vi "LCOS GUI v3_red.vi"() -> ()   [LabVIEW 2011]
uses:
  Periodic Spot Pattern Parameters.ctl
  LCOS State Machine States.ctl
  LCOS Pattern Display Actions.ctl
  LCOS Parent Action.ctl
  LCOS Images.ctl
  <vilib>/vision/Image Controls.llb/IMAQ Image.ctl
panel:
  in  "Enable Remote Control":bool=TRUE
  in  "Clear Error":bool
  in  "Ignore":bool
  out "Last Error":errorcluster
  in  "Loaded Pattern File:":bool
  out "File Path":path
  out "LCOS Pattern Preview":T1(plugin-control)
  in  "Buttons":T2={"Pattern"=enum."Computed", "Auto-Update LCOS"=TRUE, "Apply Correction"=FALSE, "Update LCOS"=FALSE, "Preview Pattern"=FALSE, "Auto-Preview"=TRUE}
  in  "Pattern Definition":T3={"X pitch"=23.0, "rotation"=0.0, "Center H"=0.0, "Center V"=0.0, "# Spots H"=5, "# Spots V"=13, "Spot size"=23.0, "ref_spot _dark"=FALSE, "Exact Phase Formula"=TRUE, "phase_wrap_pos"=FALSE, "Set Focus (mm)"=32.0, "phase_max"=4.0, "phase_factor"=60, "Steer LW"=1, "Steer vmax"=80, "phase_wrap_neg"=TRUE, "steer_horiz"=FALSE, "steer_pad"=0, "steer_only"=FALSE, "Wavelength"=6.28e-07, "Y pitch"=23.0, "python"=TRUE, "test_pattern"=FALSE, "grid"=TRUE, "dark_all"=FALSE, "Xm_str"="21.72,  44.87,  68.20,  91.45, 114.72, 137.87, 160.97, 184.04", "Ym_str"="21.72,  44.87,  68.20,  91.45, 114.72, 137.87, 160.97, 184.04", "ref_spot"=0, "stretch"=TRUE} {"ref_spot" min=0 max=500 step=1 format="%#.0f"; "Y pitch" min=0.0 max=100.0 format="%.2g"; "Wavelength" min=0.0 max=500.0 format="%^#.3e"; "steer_pad" min=0 max=500 step=1 format="%#.0f"; "Steer LW" max=500; "phase_max" min=0.0 max=500.0 format="%#.3f"; "Set Focus (mm)" min=0.0 max=500.0 format="%#.3g"; "Spot size" min=1.0 format="%.2g"; "# Spots V" min=1 step=1; "# Spots H" min=1 step=1; "Center V" format="%.2f"; "Center H" format="%.2f"; "rotation" min=-90.0 max=90.0 format="%.2g"; "X pitch" min=0.0 max=100.0 format="%.2g"}
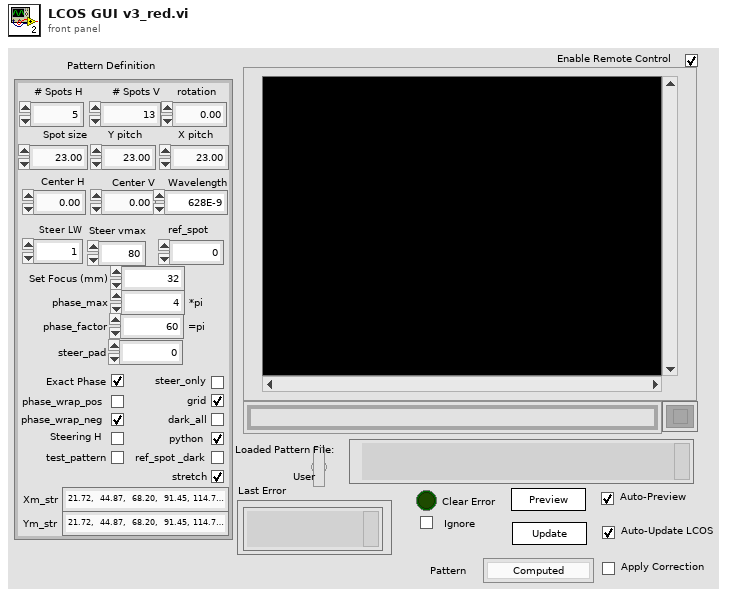
[diagram p1: front panel]
types:
  T1 = typedef "IMAQ Image.ctl" = refnum<image>
  T2 = cluster{"Pattern":enum16{"Computed", "From File", "Correction"}, "Auto-Update LCOS":bool, "Apply Correction":bool, "Update LCOS":bool, "Preview Pattern":bool, "Auto-Preview":bool}
  T3 = typedef "Periodic Spot Pattern Parameters.ctl" = cluster{"X pitch":dbl, "rotation":dbl, "Center H":dbl, "Center V":dbl, "# Spots H":u32, "# Spots V":u32, "Spot size":dbl, "ref_spot _dark":bool, "Exact Phase Formula":bool, "phase_wrap_pos":bool, "Set Focus (mm)":dbl, "phase_max":dbl, "phase_factor":u8, "Steer LW":u32, "Steer vmax":u8, "phase_wrap_neg":bool, "steer_horiz":bool, "steer_pad":i64, "steer_only":bool, "Wavelength":dbl, "Y pitch":dbl, "python":bool, "test_pattern":bool, "grid":bool, "dark_all":bool, "Xm_str":string, "Ym_str":string, "ref_spot":i64, "stretch":bool}
  T4 = typedef "LCOS Pattern Display Actions.ctl" = enum16{"Init", "Idle", "Update", "Exit"}
  T5 = cluster{"LCOS Pattern Display Actions":T4, "Data":variant}
  T6 = typedef "LCOS State Machine States.ctl" = enum16{"Init", "Idle", "Preview Button Pushed", "Update Button Pushed", "Pattern Selection Changed", "Pattern Definition Changed", "Selected File Changed", "Load Correction Pattern", "Load Correction Pattern Step 2", "Load User Pattern", "Load User Pattern Step 2", "Compute Pattern", "Correct Pattern", "Update Preview Display", "Update LCOS Display", "Error", "Clear Error", "Exit"}
  T7 = cluster{"X pitch":dbl, "rotation":dbl, "Center H":dbl, "Center V":dbl, "# Spots H":u32, "# Spots V":u32, "Spot size":dbl, "ref_spot _dark":bool, "Exact Phase Formula":bool, "phase_wrap_pos":bool, "Set Focus (mm)":dbl, "phase_max":dbl, "phase_factor":u8, "Steer LW":u32, "Steer vmax":u8, "phase_wrap_neg":bool, "steer_horiz":bool, "steer_pad":i64, "steer_only":bool, "Wavelength":dbl, "Y pitch":dbl, "python":bool, "test_pattern":bool, "grid":bool, "dark_all":bool, "Xm_str":string, "Ym_str":string, "ref_spot":i64, "stretch":bool}
  T8 = typedef "LCOS Parent Action.ctl" = enum16{"Pattern Definition Changed", "Preview Button Pushed", "Update Button Pushed", "Pattern Selection Changed", "Correction Pattern Changed", "User Pattern (from File) Changed"}
  T9 = typedef "LCOS Images.ctl" = cluster{"Computed Pattern Image":T1, "User Pattern (from File) Image":T1, "Correction Pattern Image":T1, "Corrected Pattern Image":T1, "Preview Image":T1, "LCOS Displayed Image":T1}
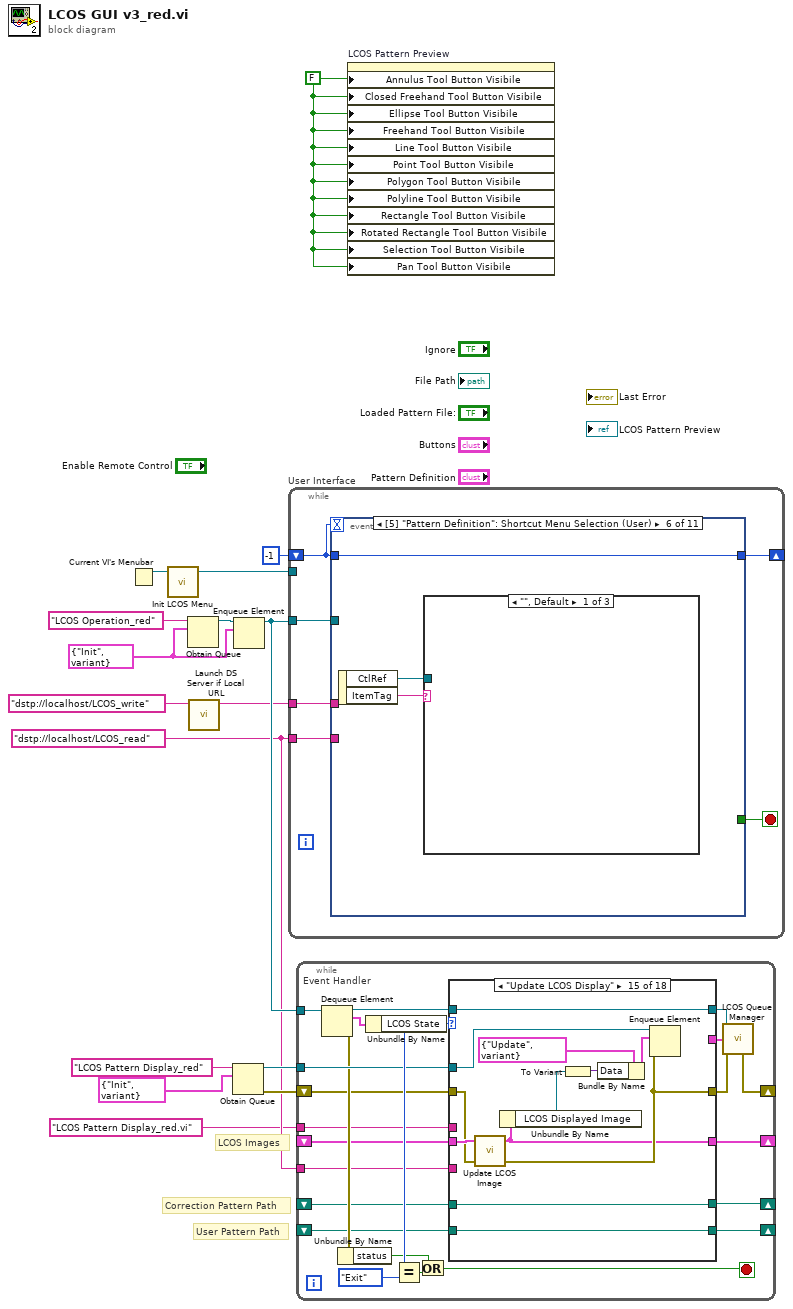
[diagram p0: block diagram]
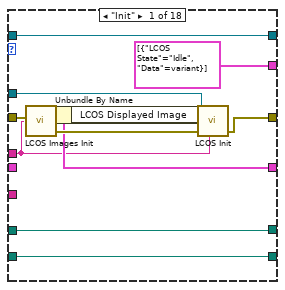
[diagram p2: hidden frame]
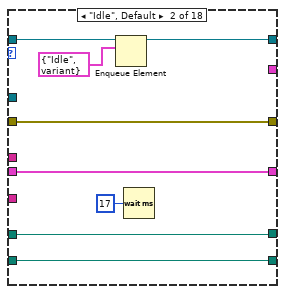
[diagram p3: hidden frame]
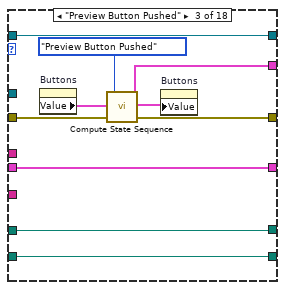
[diagram p4: hidden frame]
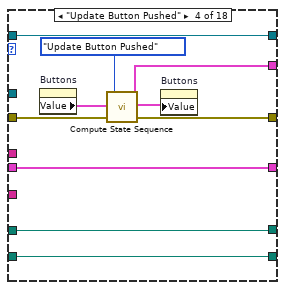
[diagram p5: hidden frame]
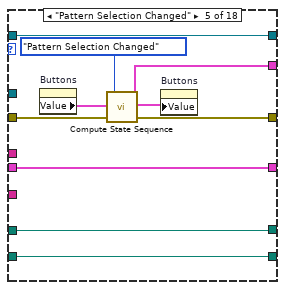
[diagram p6: hidden frame]
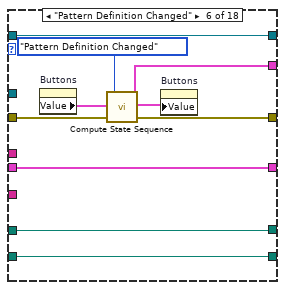
[diagram p7: hidden frame]
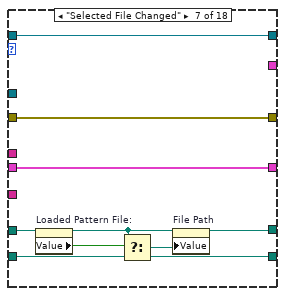
[diagram p8: hidden frame]
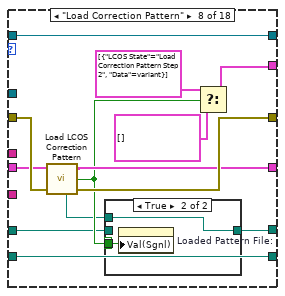
[diagram p9: hidden frame]
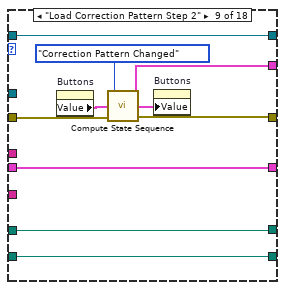
[diagram p11: hidden frame]
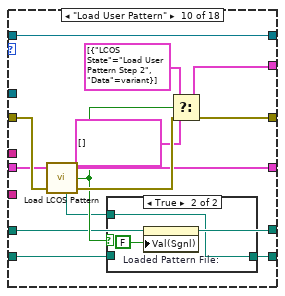
[diagram p12: hidden frame]
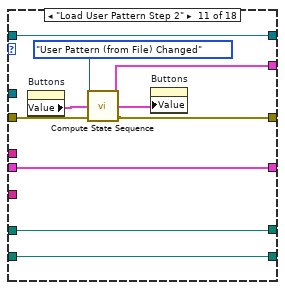
[diagram p14: hidden frame]
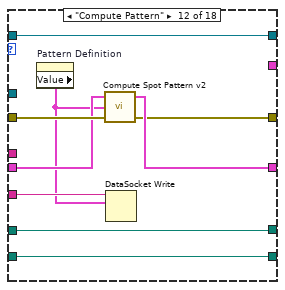
[diagram p15: hidden frame]
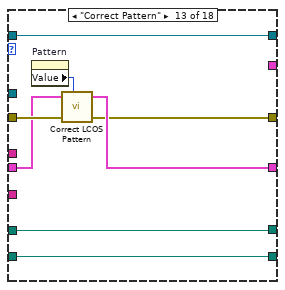
[diagram p16: hidden frame]
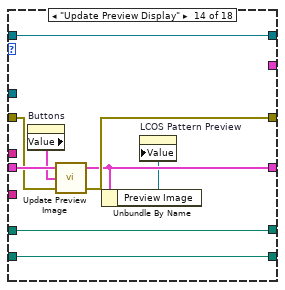
[diagram p17: hidden frame]
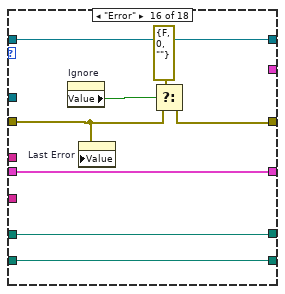
[diagram p18: hidden frame]
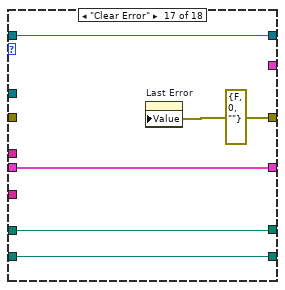
[diagram p19: hidden frame]
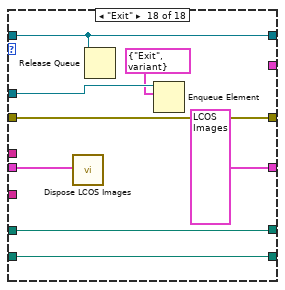
[diagram p20: hidden frame]
diagram:
  w2 = "dstp://localhost/LCOS_read" ("URL")
  w6 = FALSE ("ROI Tool Buttons Visibile:Annulus Tool Button Visibile")
  w7 = cluster{"LCOS State":T6, "Data":variant} {"LCOS State"=enum."Init", "Data"=variant}
  # "User Pattern Path"
  # "Correction Pattern Path"
  # "LCOS Images"
  n1 = Current VI's Menubar() -> (w16:refnum<k9>)
  n2 = call "Init LCOS Menu.vi"("Menu Refnum (in)"=w16) -> ("Menu Refnum (out)"=w15:refnum<k9>)  [unwired: 7 in, 1 out]
  n3 = Obtain Queue(name (unnamed)="LCOS Operation_red", element data type=w7) -> (queue out=w9:refnum<queue>)  [unwired: 3 in, 2 out]
  n4 = call "Launch DS Server if Local URL.vi"("URL"="dstp://localhost/LCOS_write") -> ("Duplicate URL"=w3:string)  [unwired: 5 in, 1 out]
  n5 = Obtain Queue(name (unnamed)="LCOS Pattern Display_red", element data type=T5 {"LCOS Pattern Display Actions"=enum."Init", "Data"=variant}) -> (queue out=w11:refnum<queue>, error out=w10:errorcluster)  [unwired: 3 in, 1 out]
  n6 = Enqueue Element(queue=w9, element=w7) -> (queue out=w8:refnum<queue>)  [unwired: 2 in, 2 out]
  n7 = while "User Interface" {
    tunnel: w15 -> [_]
    tunnel: w8 -> [w21]
    shift-right: [w20] -> _
    shift-left: -1 -> [w19]
    tunnel: w3 -> [w18]
    tunnel: w2 -> [w17]
    stop <- w22 stop-if-true
    n8 = event shown="[5] \"Pattern Definition\": Shortcut Menu Selection (User)" {
      selector: _ -> [_ _ _ _ _ _ _ _ _ _ _]
      dyn-events: _ -> [_ _ _ _ _ _ _ _ _ _ _]
      timeout: w19 -> [_ _ _ _ _ _ _ _ _ _ _]
      tunnel: [_ _ _ _ _ _ _ _ _ w63 w81] -> w22
      tunnel: w21 -> [_ _ w41 w44 w47 _ w55 w58 w61 w64 w80]
      tunnel: [w23 w35 w39 w42 w45 w50 w53 w56 w59 w62 w78] -> w20
      tunnel: w19 -> [w23 _ w39 w42 w45 w50 w53 w56 w59 w62 w78]
      tunnel: w18 -> [w28 _ _ _ _ _ _ _ _ _ _]
      tunnel: w17 -> [w24 w32 _ _ _ _ _ _ _ _ _]
      event Timeout {
        n9 = event-data() -> ()  [unwired: 1 in, 1 out]
        n10 = DataSocket Read(9:w23, 10:T3 {"X pitch"=0.0, "rotation"=0.0, "Center H"=0.0, "Center V"=0.0, "# Spots H"=0, "# Spots V"=0, "Spot size"=0.0, "ref_spot _dark"=FALSE, "Exact Phase Formula"=FALSE, "phase_wrap_pos"=FALSE, "Set Focus (mm)"=0.0, "phase_max"=0.0, "phase_factor"=0, "Steer LW"=0, "Steer vmax"=0, "phase_wrap_neg"=FALSE, "steer_horiz"=FALSE, "steer_pad"=0, "steer_only"=FALSE, "Wavelength"=0.0, "Y pitch"=0.0, "python"=FALSE, "test_pattern"=FALSE, "grid"=FALSE, "dark_all"=FALSE, "Xm_str"="", "Ym_str"="", "ref_spot"=0, "stretch"=FALSE} ("Pattern Definition"), 11:w28) -> (1:w26:bool, 2:w25:T3)  [unwired: 2 in, 5 out]
        n11 = case shown="False" w26 {
          tunnel: w25 -> [w30 _]
          tunnel: w24 -> [w31 _]
          tunnel: w23 -> [w29 _]
          frame False {
            n12 = property on="Pattern Definition" class="Clust (strict)"("Val(Sgnl)"=w30) -> ()  [unwired: 2 in, 2 out]
            n13 = DataSocket Write(9:w29, 10:w30, 11:w31) -> ()  [unwired: 1 in, 3 out]
          }
          frame True {
          }
        }
      }
      event "Enable Remote Control": Value Change {
        n14 = event-data() -> ("NewVal"=w33:bool)  [unwired: 1 in]
        n15 = case shown="False" w33 {
          tunnel: w32 -> [_ w38]
          frame False {
          }
          frame True {
            n16 = property on="Pattern Definition" class="Clust (strict)"() -> ("Value"=w37:T7)  [unwired: 2 in, 2 out]
            n17 = DataSocket Write(10:w37, 11:w38) -> ()  [unwired: 2 in, 3 out]
          }
        }
        n18 = Select(t=1, s=w33, f=-1) -> (s? t:f=w35:i32)
      }
      event Value Change {
        n19 = event-data() -> ()  [unwired: 1 in, 1 out]
        n20 = Enqueue Element(queue=w41, element=cluster{"LCOS State":T6, "Data":variant} {"LCOS State"=enum."Pattern Definition Changed", "Data"=variant}) -> ()  [unwired: 2 in, 3 out]
      }
      event "Buttons.Preview Pattern": Value Change {
        n21 = event-data() -> ()  [unwired: 1 in, 1 out]
        n22 = Enqueue Element(queue=w44, element=cluster{"LCOS State":T6, "Data":variant} {"LCOS State"=enum."Preview Button Pushed", "Data"=variant}) -> ()  [unwired: 2 in, 3 out]
      }
      event "Buttons.Update LCOS": Value Change {
        n23 = event-data() -> ()  [unwired: 1 in, 1 out]
        n24 = Enqueue Element(queue=w47, element=cluster{"LCOS State":T6, "Data":variant} {"LCOS State"=enum."Update Button Pushed", "Data"=variant}) -> ()  [unwired: 2 in, 3 out]
      }
      event Shortcut Menu Selection (User) {
        n25 = event-data() -> ("CtlRef"=w48:refnum<vi>, "ItemTag"=w49:string)  [unwired: 1 in]
        n26 = case shown="\"\", Default" w49 {
          tunnel: w48 -> [_ w51 w52]
          frame "", Default {
          }
          frame "Save Configuration" {
            n27 = call "Save LCOS Configuration.vi"("LCOS Configuration Ref"=w51) -> ()  [unwired: 11 in]
          }
          frame "Load Configuration" {
            n28 = call "Load LCOS Configuration.vi"("LCOS Configuration Ref"=w52) -> ()  [unwired: 11 in]
          }
        }
      }
      event "Buttons.Pattern": Value Change {
        n29 = event-data() -> ()  [unwired: 1 in, 4 out]
        n30 = Enqueue Element(queue=w55, element=cluster{"LCOS State":T6, "Data":variant} {"LCOS State"=enum."Pattern Selection Changed", "Data"=variant}) -> ()  [unwired: 2 in, 3 out]
      }
      event "Clear Error": Value Change {
        n31 = event-data() -> ()  [unwired: 1 in, 1 out]
        n32 = Enqueue Element(queue=w58, element=cluster{"LCOS State":T6, "Data":variant} {"LCOS State"=enum."Clear Error", "Data"=variant}) -> ()  [unwired: 2 in, 3 out]
      }
      event "Loaded Pattern File:": Value Change {
        n33 = event-data() -> ()  [unwired: 1 in, 1 out]
        n34 = Enqueue Element(queue=w61, element=cluster{"LCOS State":T6, "Data":variant} {"LCOS State"=enum."Selected File Changed", "Data"=variant}) -> ()  [unwired: 2 in, 3 out]
      }
      event Menu Selection (User) {
        n35 = event-data() -> ("ItemTag"=w65:string)  [unwired: 1 in]
        n36 = case shown="\"Load Correction Pattern\"" w65 {
          tunnel: w64 -> [_ w67 w69 w73]
          tunnel: [_ _ _ w70] -> w63
          frame "-", Default {
          }
          frame "Load Correction Pattern" {
            n37 = Enqueue Element(queue=w67, element=cluster{"LCOS State":T6, "Data":variant} {"LCOS State"=enum."Load Correction Pattern", "Data"=variant}) -> ()  [unwired: 2 in, 3 out]
          }
          frame "Load User Pattern" {
            n38 = Enqueue Element(queue=w69, element=cluster{"LCOS State":T6, "Data":variant} {"LCOS State"=enum."Load User Pattern", "Data"=variant}) -> ()  [unwired: 2 in, 3 out]
          }
          frame "Quit" {
            n39 = Two Button Dialog(message="Do you want to quit?") -> (T button?=w70:bool)  [unwired: 2 in]
            n40 = case shown="True" w70 {
              tunnel: w73 -> [w74 w77]
              tunnel: [w74 w76] -> _
              tunnel: cluster{"LCOS State":T6, "Data":variant} {"LCOS State"=enum."Exit", "Data"=variant} ("element") -> [_ w75]
              frame False {
              }
              frame True {
                n41 = Enqueue Element(queue=w77, element=w75) -> (queue out=w76:refnum<queue>)  [unwired: 2 in, 2 out]
              }
            }
          }
        }
      }
      event Panel Close? {
        w81 = TRUE ("Discard?")
        n42 = event-data() -> ()  [unwired: 1 in, 1 out]
        n43 = Enqueue Element(queue=w80, element=cluster{"LCOS State":T6, "Data":variant} {"LCOS State"=enum."Exit", "Data"=variant}) -> ()  [unwired: 2 in, 3 out]
        n44 = event-data("Discard?"=w81) -> ()  [unwired: 1 in, 1 out]
      }
    }
  }
  n45 = while "Event Handler" {
    tunnel: w11 -> [w99]
    shift-right: [w93] -> _
    shift-left: w10 -> [w91]
    tunnel: w8 -> [w104]
    shift-right: [w89] -> _
    shift-left: _ -> [w90]
    shift-right: [w87] -> _
    shift-left: _ -> [w86]
    shift-right: [w85] -> _
    shift-left: _ -> [w84]
    tunnel: w2 -> [w83]
    tunnel: "LCOS Pattern Display_red.vi" ("name (unnamed)") -> [w82]
    stop <- w96 stop-if-true
    n46 = Dequeue Element(queue=w104) -> (queue out=w100:refnum<queue>, element=w98:cluster{"LCOS State":T6, "Data":variant}, error out=w97:errorcluster)  [unwired: 2 in, 1 out]
    n47 = Unbundle By Name(w97) -> ("status"=w95:bool)
    n48 = Unbundle By Name(w98) -> ("LCOS State"=w103:T6)
    n49 = Equal?(x=w103, y=LCOS_State_Machine_States."Exit") -> (x = y?=w101:bool)
    n50 = Or(x=w95, y=w101) -> (x .or. y?=w96:bool)
    n51 = case shown="\"Update LCOS Display\"" w103 {
      tunnel: w100 -> [w108 w123 w130 w140 w150 w160 w170 w178 w194 w204 w220 w227 w234 w248 w256 w263 w271 w276]
      tunnel: w99 -> [w115 _ _ _ _ _ _ _ _ _ _ _ _ _ w260 _ _ w280]
      tunnel: [cluster{"LCOS State":T6, "Data":variant}[] [{"LCOS State"=enum."Idle", "Data"=variant}] ("Action Sequence") _ w127 w137 w147 w157 _ w181 w191 w206 w217 _ _ _ _ _ _ _] -> w94
      tunnel: [w114 w121 w128 w138 w148 w158 w169 w182 w192 w208 w218 w228 w235 w244 w253 w266 w273 w281] -> w92
      tunnel: w91 -> [w113 w121 w129 w139 w149 w159 w169 w183 w193 w209 w219 w231 w238 w245 w254 w264 _ w281]
      tunnel: w90 -> [_ w119 w132 w142 w152 w162 w168 w177 w189 w203 w215 w230 w237 w247 w255 w268 w272 w278]
      tunnel: [w110 w119 w132 w142 w152 w162 w168 w176 w189 w202 w215 w229 w236 w243 w252 w268 w272 T9 {"Computed Pattern Image"=refnum, "User Pattern (from File) Image"=refnum, "Correction Pattern Image"=refnum, "Corrected Pattern Image"=refnum, "Preview Image"=refnum, "LCOS Displayed Image"=refnum} ("Images")] -> w89
      tunnel: [w108 w118 w130 w140 w150 w160 w170 w178 w194 w204 w220 w227 w234 w248 w256 w263 w271 w276] -> w88
      tunnel: [w107 w117 w125 w135 w145 w155 w165 w173 w188 w197 w214 w226 w233 w241 w250 w262 w270 w275] -> w87
      tunnel: w86 -> [w107 w117 w125 w135 w145 w155 w165 w174 w188 w197 w214 w226 w233 w241 w250 w262 w270 w275]
      tunnel: [w106 w116 w124 w134 w144 w154 w166 w171 w187 w199 w213 w225 w232 w240 w249 w261 w269 w274] -> w85
      tunnel: w84 -> [w106 w116 w124 w134 w144 w154 w166 w171 w187 w198 w213 w225 w232 w240 w249 w261 w269 w274]
      tunnel: w83 -> [_ _ _ _ _ _ _ _ _ _ _ w224 _ _ _ _ _ _]
      tunnel: w82 -> [w105 _ _ _ _ _ _ _ _ _ _ _ _ _ _ _ _ _]
      frame "Init" {
        n52 = call "LCOS Images Init.vi"("LCOS Pattern Display.vi Name"=w105, "error in (no error)"=w113) -> ("Images"=w110:T9, "error out"=w112:errorcluster)  [unwired: 6 in]
        n53 = Unbundle By Name(w110) -> ("LCOS Displayed Image"=w111:T1)
        n54 = call "LCOS Init.vi"("LCOS Display Queue"=w115, "LCOS Displayed Image"=w111, "error in (no error)"=w112, "LCOS Pattern Display.vi Name"=w105) -> ("error out"=w114:errorcluster)  [unwired: 5 in]
      }
      frame "Idle", Default {
        n55 = Enqueue Element(queue=w123, element=cluster{"LCOS State":T6, "Data":variant} {"LCOS State"=enum."Idle", "Data"=variant}) -> (queue out=w118:refnum<queue>)  [unwired: 2 in, 2 out]
        n56 = Wait (ms)(milliseconds to wait=u32 17) -> ()  [unwired: 1 out]
      }
      frame "Preview Button Pushed" {
        n57 = property on="Buttons" class="Clust (strict)"() -> ("Value"=w133:T2)  [unwired: 2 in, 2 out]
        n58 = call "Compute State Sequence.vi"("Parent Action"=LCOS_Parent_Action."Preview Button Pushed" ("Previous Event"), "Buttons (in)"=w133, "error in (no error)"=w129) -> ("Action Sequence"=w127:cluster{"LCOS State":T6, "Data":variant}[], "Buttons (out)"=w126:T2, "error out"=w128:errorcluster)  [unwired: 4 in]
        n59 = property on="Buttons" class="Clust (strict)"("Value"=w126) -> ()  [unwired: 2 in, 2 out]
      }
      frame "Update Button Pushed" {
        n60 = property on="Buttons" class="Clust (strict)"() -> ("Value"=w143:T2)  [unwired: 2 in, 2 out]
        n61 = call "Compute State Sequence.vi"("Parent Action"=LCOS_Parent_Action."Update Button Pushed" ("Previous Event"), "Buttons (in)"=w143, "error in (no error)"=w139) -> ("Action Sequence"=w137:cluster{"LCOS State":T6, "Data":variant}[], "Buttons (out)"=w136:T2, "error out"=w138:errorcluster)  [unwired: 4 in]
        n62 = property on="Buttons" class="Clust (strict)"("Value"=w136) -> ()  [unwired: 2 in, 2 out]
      }
      frame "Pattern Selection Changed" {
        n63 = property on="Buttons" class="Clust (strict)"() -> ("Value"=w153:T2)  [unwired: 2 in, 2 out]
        n64 = call "Compute State Sequence.vi"("Parent Action"=LCOS_Parent_Action."Pattern Selection Changed" ("Previous Event"), "Buttons (in)"=w153, "error in (no error)"=w149) -> ("Action Sequence"=w147:cluster{"LCOS State":T6, "Data":variant}[], "Buttons (out)"=w146:T2, "error out"=w148:errorcluster)  [unwired: 4 in]
        n65 = property on="Buttons" class="Clust (strict)"("Value"=w146) -> ()  [unwired: 2 in, 2 out]
      }
      frame "Pattern Definition Changed" {
        n66 = property on="Buttons" class="Clust (strict)"() -> ("Value"=w163:T2)  [unwired: 2 in, 2 out]
        n67 = call "Compute State Sequence.vi"("Parent Action"=LCOS_Parent_Action."Pattern Definition Changed" ("Previous Event"), "Buttons (in)"=w163, "error in (no error)"=w159) -> ("Action Sequence"=w157:cluster{"LCOS State":T6, "Data":variant}[], "Buttons (out)"=w156:T2, "error out"=w158:errorcluster)  [unwired: 4 in]
        n68 = property on="Buttons" class="Clust (strict)"("Value"=w156) -> ()  [unwired: 2 in, 2 out]
      }
      frame "Selected File Changed" {
        n69 = property on="Loaded Pattern File:" class="Bool (strict)"() -> ("Value"=w167:bool)  [unwired: 2 in, 2 out]
        n70 = Select(t=w165, s=w167, f=w166) -> (s? t:f=w164:path)
        n71 = property on="File Path" class="Path"("Value"=w164) -> ()  [unwired: 2 in, 2 out]
      }
      frame "Load Correction Pattern" {
        n72 = call "Load LCOS Correction Pattern.vi"("Images Dest"=w177, "error in"=w183) -> ("Images Out"=w176:T9, "Correct File Type"=w175:bool, "Path"=w172:path, "error out"=w182:errorcluster)  [unwired: 3 in, 1 out]
        n73 = case shown="True" w175 {
          tunnel: w175 -> [_ w186]
          tunnel: w174 -> [w184 _]
          tunnel: [w184 w185] -> w173
          tunnel: w172 -> [_ w185]
          frame False {
          }
          frame True {
            n74 = property on="Loaded Pattern File:" class="Bool (strict)"("Val(Sgnl)"=w186) -> ()  [unwired: 2 in, 2 out]
          }
        }
        n75 = Select(t=cluster{"LCOS State":T6, "Data":variant}[] [{"LCOS State"=enum."Load Correction Pattern Step 2", "Data"=variant}], s=w175, f=cluster{"LCOS State":T6, "Data":variant}[] []) -> (s? t:f=w181:cluster{"LCOS State":T6, "Data":variant}[])
      }
      frame "Load Correction Pattern Step 2" {
        n76 = property on="Buttons" class="Clust (strict)"() -> ("Value"=w196:T2)  [unwired: 2 in, 2 out]
        n77 = call "Compute State Sequence.vi"("Parent Action"=LCOS_Parent_Action."Correction Pattern Changed" ("Previous Event"), "Buttons (in)"=w196, "error in (no error)"=w193) -> ("Action Sequence"=w191:cluster{"LCOS State":T6, "Data":variant}[], "Buttons (out)"=w190:T2, "error out"=w192:errorcluster)  [unwired: 4 in]
        n78 = property on="Buttons" class="Clust (strict)"("Value"=w190) -> ()  [unwired: 2 in, 2 out]
      }
      frame "Load User Pattern" {
        n79 = call "Load LCOS Pattern.vi"("Images Dest"=w203, "error in"=w209) -> ("Images Out"=w202:T9, "Correct File Type"=w201:bool, "Path"=w200:path, "error out"=w208:errorcluster)  [unwired: 3 in, 1 out]
        n80 = case shown="True" w201 {
          tunnel: w198 -> [w210 _]
          tunnel: [w210 w212] -> w199
          tunnel: w200 -> [_ w212]
          frame False {
          }
          frame True {
            n81 = property on="Loaded Pattern File:" class="Bool (strict)"("Val(Sgnl)"=FALSE ("Value (Signaling)")) -> ()  [unwired: 2 in, 2 out]
          }
        }
        n82 = Select(t=cluster{"LCOS State":T6, "Data":variant}[] [{"LCOS State"=enum."Load User Pattern Step 2", "Data"=variant}], s=w201, f=cluster{"LCOS State":T6, "Data":variant}[] []) -> (s? t:f=w206:cluster{"LCOS State":T6, "Data":variant}[])
      }
      frame "Load User Pattern Step 2" {
        n83 = property on="Buttons" class="Clust (strict)"() -> ("Value"=w222:T2)  [unwired: 2 in, 2 out]
        n84 = call "Compute State Sequence.vi"("Parent Action"=LCOS_Parent_Action."User Pattern (from File) Changed" ("Previous Event"), "Buttons (in)"=w222, "error in (no error)"=w219) -> ("Action Sequence"=w217:cluster{"LCOS State":T6, "Data":variant}[], "Buttons (out)"=w216:T2, "error out"=w218:errorcluster)  [unwired: 4 in]
        n85 = property on="Buttons" class="Clust (strict)"("Value"=w216) -> ()  [unwired: 2 in, 2 out]
      }
      frame "Compute Pattern" {
        n86 = property on="Pattern Definition" class="Clust (strict)"() -> ("Value"=w223:T7)  [unwired: 2 in, 2 out]
        n87 = call "Compute Spot Pattern v2.vi"("Images Dest"=w230, "Pattern Definition"=w223, "error in"=w231) -> ("Images Out"=w229:T9, "error out"=w228:errorcluster)  [unwired: 3 in, 2 out]
        n88 = DataSocket Write(10:w223, 11:w224) -> ()  [unwired: 2 in, 3 out]
      }
      frame "Correct Pattern" {
        n89 = property on="Pattern" class="Enum (strict)"() -> ("Value"=w239:enum16{"Computed", "From File", "Correction"})  [unwired: 2 in, 2 out]
        n90 = call "Correct LCOS Pattern.vi"("Images Dest"=w237, "Pattern"=w239, "error in"=w238) -> ("Images Out"=w236:T9, "error out"=w235:errorcluster)  [unwired: 5 in]
      }
      frame "Update Preview Display" {
        n91 = property on="Buttons" class="Clust (strict)"() -> ("Value"=w246:T2)  [unwired: 2 in, 2 out]
        n92 = call "Update Preview Image.vi"("Images (Dest)"=w247, "Buttons"=w246, "error in"=w245) -> ("Images (Out)"=w243:T9, "error out"=w244:errorcluster)  [unwired: 5 in]
        n93 = Unbundle By Name(w243) -> ("Preview Image"=w242:T1)
        n94 = property on="LCOS Pattern Preview" class="ImageControl"("Value"=w242) -> ()  [unwired: 2 in, 2 out]
      }
      frame "Update LCOS Display" {
        n95 = call "Update LCOS Image.vi"("Images (Dest)"=w255, "error in"=w254) -> ("Images (Out)"=w252:T9, "error out"=w253:errorcluster)  [unwired: 6 in]
        n96 = Unbundle By Name(w252) -> ("LCOS Displayed Image"=w251:T1)
        n97 = To Variant(anything=w251) -> (Variant=w257:variant)
        n98 = Bundle By Name(cluster=T5 {"LCOS Pattern Display Actions"=enum."Update", "Data"=variant}, "Data"=w257) -> (w258:T5)
        n99 = Enqueue Element(queue=w260, element=w258, error in (no error)=w253) -> ()  [unwired: 1 in, 3 out]
      }
      frame "Error" {
        n100 = property on="Ignore" class="Bool (strict)"() -> ("Value"=w267:bool)  [unwired: 2 in, 2 out]
        n101 = property on="Last Error" class="Clust (strict)"("Value"=w264) -> ()  [unwired: 2 in, 2 out]
        n102 = Select(t=errorcluster {"status"=FALSE, "code"=0, "source"=""}, s=w267, f=w264) -> (s? t:f=w266:errorcluster)
      }
      frame "Clear Error" {
        w273 = errorcluster {"status"=FALSE, "code"=0, "source"=""} ("error out")
        n103 = property on="Last Error" class="Clust (strict)"("Value"=w273) -> ()  [unwired: 2 in, 2 out]
      }
      frame "Exit" {
        n104 = call "Dispose LCOS Images.vi"("Images"=w278) -> ()
        n105 = Release Queue(queue=w276) -> ()  [unwired: 2 in, 3 out]
        n106 = Enqueue Element(queue=w280, element=T5 {"LCOS Pattern Display Actions"=enum."Exit", "Data"=variant}) -> ()  [unwired: 2 in, 3 out]
      }
    }
    n107 = call "LCOS Queue Manager.vi"("Queue"=w88, "Queue States"=w94, "error in (no error)"=w92) -> ("error out"=w93:errorcluster)  [unwired: 6 in]
  }
  n108 = property on="LCOS Pattern Preview" class="ImageControl"("Annulus Tool Button Visibile"=w6, "Closed Freehand Tool Button Visibile"=w6, "Ellipse Tool Button Visibile"=w6, "Freehand Tool Button Visibile"=w6, "Line Tool Button Visibile"=w6, "Point Tool Button Visibile"=w6, "Polygon Tool Button Visibile"=w6, "Polyline Tool Button Visibile"=w6, "Rectangle Tool Button Visibile"=w6, "Rotated Rectangle Tool Button Visibile"=w6, "Selection Tool Button Visibile"=w6, "Pan Tool Button Visibile"=w6) -> ()  [unwired: 2 in, 2 out]
